vi "GUItoPLCBoolArray.vi"(11 "Input Array":bool[](array[boolean])) -> (3 "DB Array":u8[](array[numeric]))   [LabVIEW 2023]
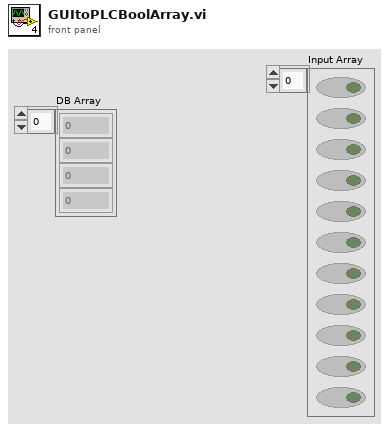
[diagram p1: front panel]
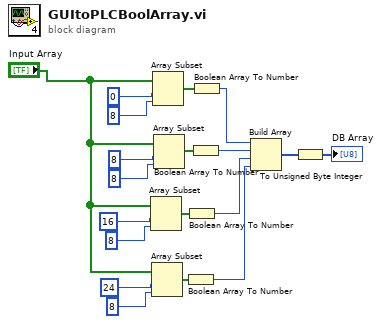
[diagram p0: block diagram]
diagram:
  n1 = Array Subset(array="Input Array", index=16, length=8) -> (w9:bool[])
  n2 = Array Subset(array="Input Array", index=24, length=8) -> (w10:bool[])
  n3 = Array Subset(array="Input Array", index=0, length=8) -> (w7:bool[])
  n4 = Array Subset(array="Input Array", index=8, length=8) -> (w8:bool[])
  n5 = Boolean Array To Number(Boolean array=w10) -> (number=w3:u32)
  n6 = Boolean Array To Number(Boolean array=w9) -> (number=w4:u32)
  n7 = Boolean Array To Number(Boolean array=w8) -> (number=w5:u32)
  n8 = Boolean Array To Number(Boolean array=w7) -> (number=w6:u32)
  n9 = Build Array(w6, w5, w4, w3) -> (w2:u32[])
  n10 = To Unsigned Byte Integer(number=w2) -> (unsigned 8bit integer=→"DB Array":u8[])
